vi "Interfaz de caracterizaçao.vi"() -> ()   [LabVIEW 2015]
uses:
  <vilib>/Analysis/baseanly.llb/Mean (DBL).vi
  <instrlib>/Agilent E364X Series/Agilent E364X Series.lvlib
  <instrlib>/Agilent 428X Series/Agilent 428X Series.lvlib
  <vilib>/Analysis/NI_AALBase.lvlib
panel:
  out "Fita2":bool
  out "Fita1":bool
  in  "Passo":dbl=0.01
  out "Fase Med":dbl format="%^.4e"
  in  "Faixa":dbl=2.0
  out "Level":dbl
  out "Config total GA":dbl[](array[numeric])
  out "Final Stop":bool
  in  "error in (no error)":errorcluster
  in  "RLC port":refnum<visa-resource-name>="GPIB0::17::INSTR"
  out "Configuração GA":dbl[](array[numeric])
  out "Otimos":dbl[](array[numeric])
  out "S_ot":dbl
  in  "milliseconds to wait":u32=1000
  out "Returned Data":string
  out "Frec OPT":dbl
  out "H(Oe) OPT":dbl
  out "Bias current OPT":dbl
  out "todo":dbl[](array[numeric])
  out "element":dbl
  out "Iteraciones":i32
  out "Corrente":dbl
  out "RELE 2":bool
  out "Modulo 2":cluster{"X":dbl[], "Y":dbl[]}[](graph) caption="XY Graph"
  out "Fase 2":cluster{"X":dbl[], "Y":dbl[]}[](graph) caption="XY Graph"
  out "Fase":dbl format="%^.4e"
  out "Modulo":dbl format="%^.4e"
  out "Data Status 2":bool=TRUE
  in  "Voltage (V)(1.0V) 2":dbl=1.0 min=0.0 max=20.0 step=0.1 format="%.4f"
  in  "Imp Type (0: CPD)":u32(ring)=15 items=["CPD", "CPQ", "CPG", "CPRP", "CSD", "CSQ", "CSRS", "LPQ", "LPD", "LPG", "LPRP", "LSD", "LSQ", "LSRS", "RX", "ZTD", "ZTR", "GB", "YTD", "YTR"]
  in  "RLC port 2":refnum<visa-resource-name>="GPIB0::17::INSTR"
  in  "error in (no error) 2":errorcluster
  out "RELE":bool
  out "Current Value":dbl
  out "Data Status":bool=TRUE
  in  "Voltage (V)(1.0V)":dbl=1.0 min=0.0 max=20.0 step=0.1 format="%.4f"
  out "Data to MatLab":dbl[](array[numeric])
  out "Data from MatLab":dbl[](array[numeric]) format="%.6g"
  # "Optimization"
  # "Characterization"
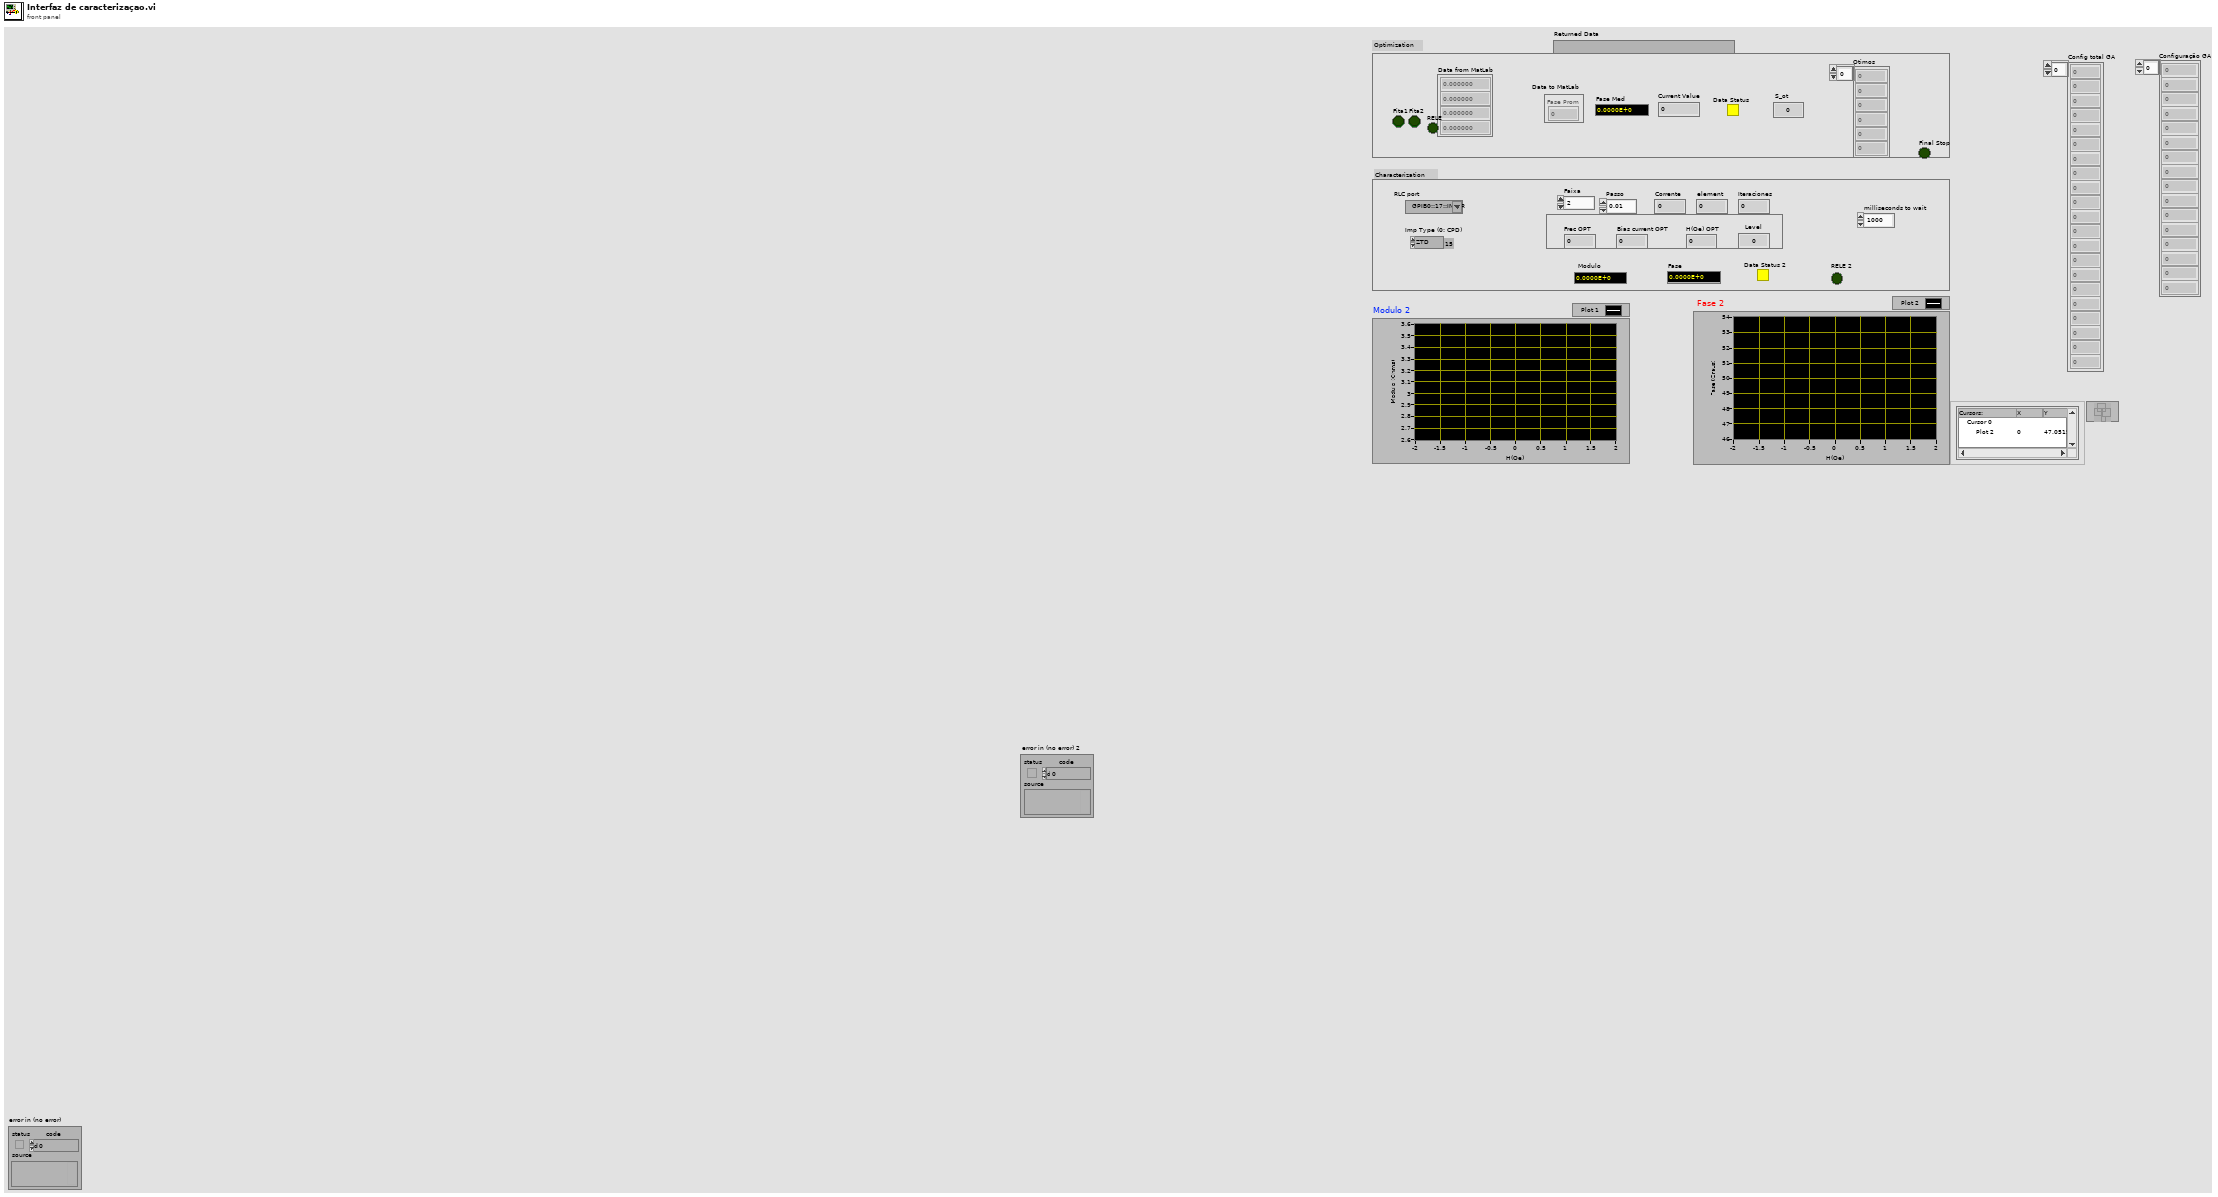
[diagram p1: front panel]
types:
  T1 = enum16{"Standard", "Buffered", "CRLF", "Immediate"}
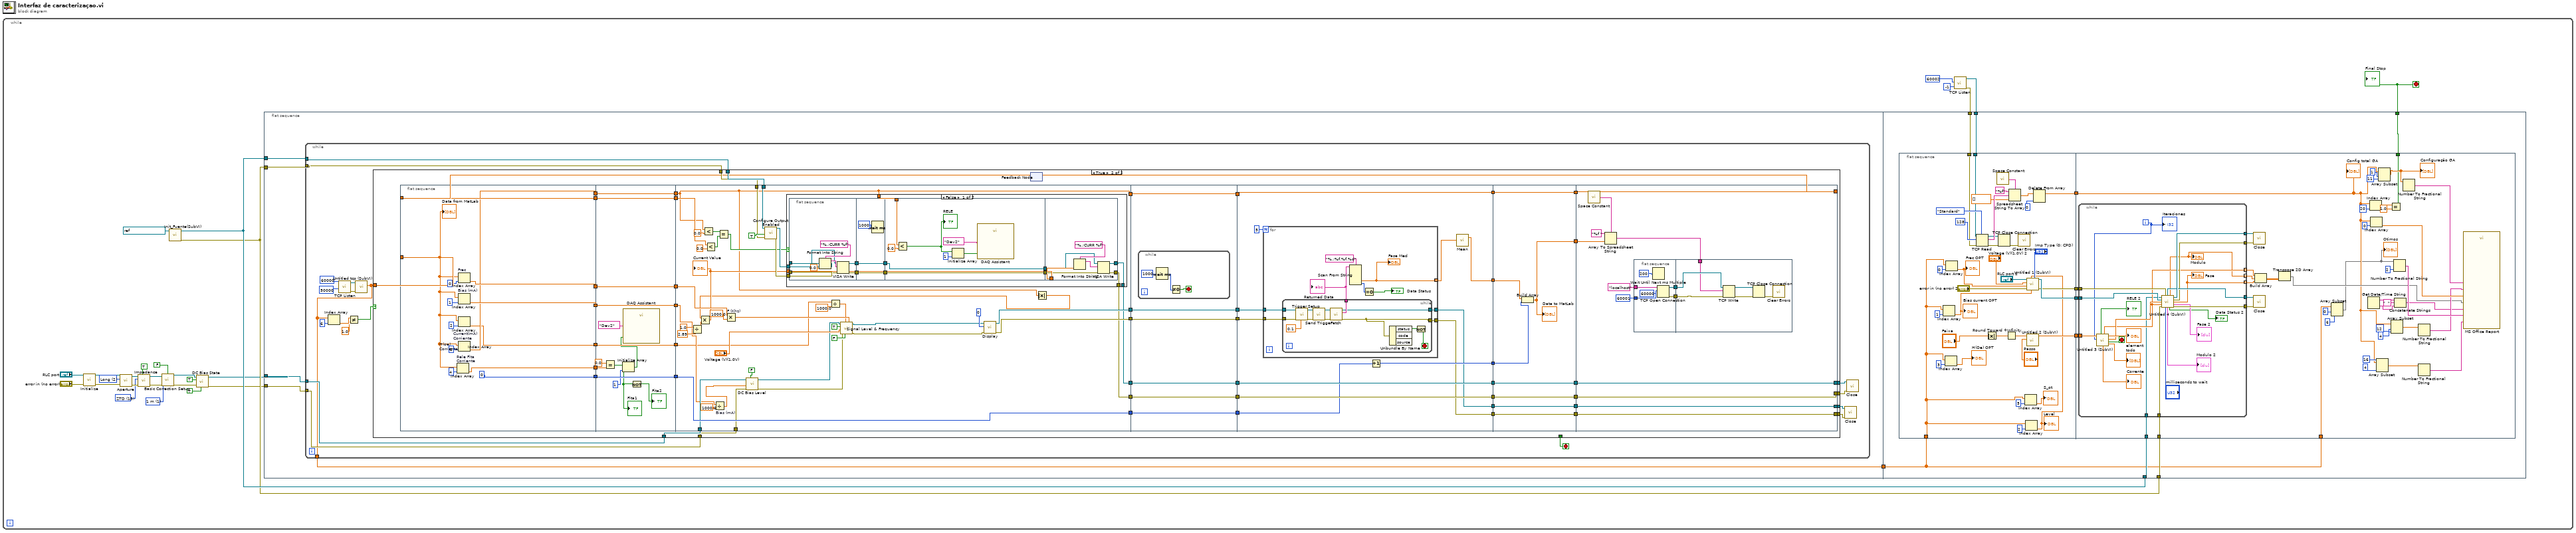
[diagram p0: block diagram]
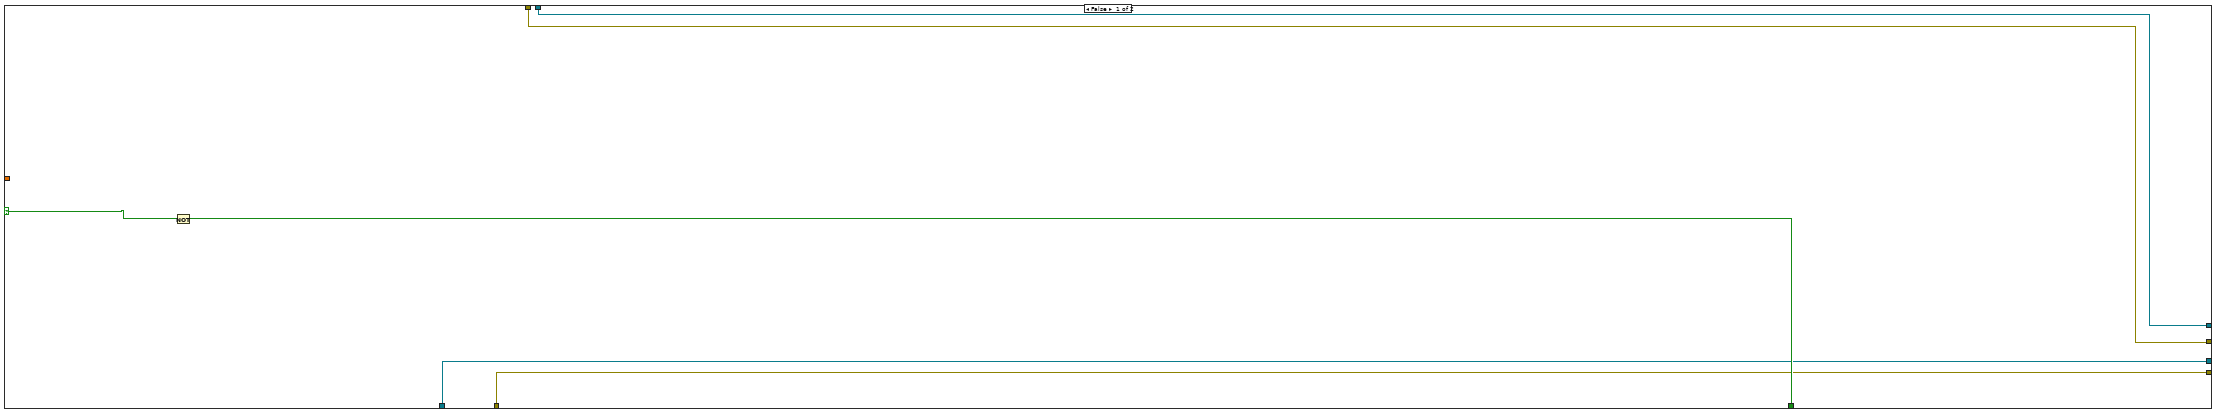
[diagram p2: hidden frame]
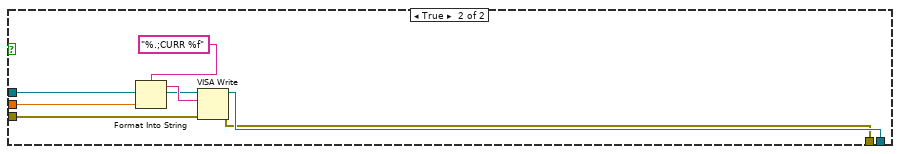
[diagram p3: hidden frame]
diagram:
  n1 = while {
    stop <- w2 stop-if-true
    w13 = u32 1 items=["0 m", "1 m", "2 m", "3 m", "4 m"] ("Cable Length (0: 4 m)")
    w20 = u32 15 items=["CPD", "CPQ", "CPG", "CPRP", "CSD", "CSQ", "CSRS", "LPQ", "LPD", "LPG", "LPRP", "LSD", "LSQ", "LSRS", "RX", "ZTD", "ZTR", "GB", "YTD", "YTR"] ("Imp Type (0: CPD)")
    w24 = u32 2 items=["Short", "Medium", "Long"] ("Integ Time (0: Short)")
    n2 = call <instrlib>:"Initialize.vi"("error in (no error)"="error in (no error)", "VISA resource name"="RLC port") -> ("error out"=w25:errorcluster, "VISA resource name out"=w26:refnum<visa-resource-name>)  [unwired: 8 in]
    n3 = call <instrlib>:"Aperture.vi"("error in (no error)"=w25, "Integ Time (0: Short)"=w24, "VISA resource name"=w26) -> ("error out"=w23:errorcluster, "VISA resource name out"=w22:refnum<visa-resource-name>)  [unwired: 7 in]
    n4 = call <instrlib>:"Impedance.vi"("Auto Range (F: Off)"=TRUE, "error in (no error)"=w23, "Imp Type (0: CPD)"=w20, "VISA resource name"=w22) -> ("error out"=w15:errorcluster, "VISA resource name out"=w17:refnum<visa-resource-name>)  [unwired: 6 in]
    n5 = call <instrlib>:"Basic Correction Setup.vi"("VISA resource name"=w17, "Short Corr (T: On)"=FALSE, "Cable Length (0: 4 m)"=w13, "error in (no error)"=w15) -> ("VISA resource name out"=w16:refnum<visa-resource-name>, "error out"=w14:errorcluster)  [unwired: 9 in, 1 out]
    n6 = call "Init_Fuente(SubVI).vi"("VISA Refnum in"=refnum<visa-resource-name> "GPIB0::5::INSTR") -> ("error out"=w9:errorcluster, "VISA Refnum out"=w10:refnum<visa-resource-name>)  [unwired: 9 in]
    n7 = call <instrlib>:"DC Bias State.vi"("Curr Bias Monitor (F: Off)"=TRUE, "error in (no error)"=w14, "State (F: Off)"=TRUE, "VISA resource name"=w16) -> ("error out"=w7:errorcluster, "VISA resource name out"=w8:refnum<visa-resource-name>)  [unwired: 6 in]
    n8 = flat-sequence {
      tunnel: w10 -> [w33]
      tunnel: w9 -> [w32]
      tunnel: w8 -> [w31]
      tunnel: w7 -> [w30]
      tunnel: [w29] -> w1
      tunnel: w10 -> [w300]
      tunnel: w9 -> [w299]
      tunnel: w4 -> [w297]
      tunnel: w3 -> [w296]
      tunnel: [w295] -> w2
      tunnel: w1 -> [w294]
      frame #0 {
        n9 = while {
          tunnel: w33 -> [w49]
          tunnel: w32 -> [w48]
          tunnel: w31 -> [w51]
          tunnel: w30 -> [w50]
          tunnel: [w38] -> w29
          stop <- w39 stop-if-true
          n10 = call <vilib>:"TCP Listen.vi"("timeout ms (wait forever: -1)"=50000, "port"=u16 60000) -> ("error out"=w44:errorcluster, "connection ID"=w45:refnum<k5>)  [unwired: 5 in, 3 out]
          n11 = call "Untitled tcp (SubVI).vi"("error in (no error)"=w44, "TCP Network Connection in"=w45) -> ("array type (2D Dbl)"=w38:dbl[])  [unwired: 7 in, 2 out]
          n12 = Index Array(array=w38, index=6) -> (element=w42:dbl)
          n13 = Not Equal?(x=w42, y=1.0) -> (x != y?=w40:bool)
          n14 = case shown="True" w40 {
            selector: w40 -> [w57 _]
            tunnel: w51 -> [w55 w81]
            tunnel: w50 -> [w54 w80]
            tunnel: w49 -> [w53 w79]
            tunnel: w48 -> [w52 w78]
            tunnel: w38 -> [_ w76]
            tunnel: [w56 _] -> w39
            tunnel: [w55 w74] -> w37
            tunnel: [w54 w73] -> w36
            tunnel: [w53 w72] -> w35
            tunnel: [w52 w71] -> w34
            frame False {
              n15 = Not(x=w57) -> (.not. x?=w56:bool)
            }
            frame True {
              n16 = flat-sequence {
                tunnel: [w115] -> w70
                tunnel: [w114] -> w68
                tunnel: [0 ("index")] -> w66
                tunnel: [w113] -> w64
                tunnel: [w116] -> w62
                tunnel: w75 -> [w116]
                tunnel: [w110] -> w60
                tunnel: w76 -> [w109]
                tunnel: [w107] -> w58
                tunnel: w70 -> [w132]
                tunnel: [w132] -> w69
                tunnel: w68 -> [w131]
                tunnel: [w131] -> w67
                tunnel: w66 -> [w130]
                tunnel: [w130] -> w65
                tunnel: w64 -> [w129]
                tunnel: [w129] -> w63
                tunnel: w62 -> [w128]
                tunnel: [w128] -> w61
                tunnel: w60 -> [w127]
                tunnel: [w127] -> w59
                tunnel: w58 -> [w126]
                tunnel: w69 -> [w170]
                tunnel: w67 -> [w145]
                tunnel: w65 -> [w162]
                tunnel: [w164] -> w106
                tunnel: [w163] -> w105
                tunnel: [w162] -> w104
                tunnel: [w161] -> w103
                tunnel: [w160] -> w102
                tunnel: w81 -> [w149]
                tunnel: w80 -> [w148]
                tunnel: w79 -> [w157]
                tunnel: w78 -> [w156]
                tunnel: w63 -> [w136]
                tunnel: [w136] -> w101
                tunnel: w61 -> [w137]
                tunnel: w59 -> [w133]
                tunnel: [w224] -> w100
                tunnel: w106 -> [w224]
                tunnel: w105 -> [w223]
                tunnel: [w223] -> w99
                tunnel: w104 -> [w222]
                tunnel: [w222] -> w98
                tunnel: [w221] -> w97
                tunnel: w103 -> [w221]
                tunnel: [w220] -> w96
                tunnel: w102 -> [w220]
                tunnel: w101 -> [w219]
                tunnel: [w219] -> w95
                tunnel: w100 -> [w239]
                tunnel: w99 -> [w228]
                tunnel: w98 -> [w235]
                tunnel: [w233] -> w94
                tunnel: [w229] -> w93
                tunnel: [w238] -> w92
                tunnel: w97 -> [w238]
                tunnel: [w237] -> w91
                tunnel: w96 -> [w237]
                tunnel: [w236] -> w90
                tunnel: [w234] -> w89
                tunnel: w95 -> [w234]
                tunnel: [w230] -> w88
                tunnel: [w268] -> w87
                tunnel: [w266] -> w86
                tunnel: w94 -> [w266]
                tunnel: [w265] -> w85
                tunnel: w93 -> [w265]
                tunnel: [w264] -> w84
                tunnel: w92 -> [w264]
                tunnel: [w263] -> w83
                tunnel: w91 -> [w263]
                tunnel: w90 -> [w262]
                tunnel: [w261] -> w82
                tunnel: w89 -> [w261]
                tunnel: w88 -> [w267]
                tunnel: w87 -> [w274]
                tunnel: [w273] -> w74
                tunnel: w86 -> [w273]
                tunnel: [w272] -> w73
                tunnel: w85 -> [w272]
                tunnel: [w271] -> w72
                tunnel: w84 -> [w271]
                tunnel: [w270] -> w71
                tunnel: w83 -> [w270]
                tunnel: [w269] -> w77
                tunnel: w82 -> [w269]
                frame #0 {
                  n17 = Index Array "Rele Fita\nCorriente"(array=w109, index=4) -> (element=w107:dbl)
                  n18 = Index Array "Frec"(array=w109, index=0) -> (element=w115:dbl)
                  n19 = Index Array "Bias (mA)"(array=w109, index=1) -> (element=w114:dbl)
                  n20 = Index Array "H(oe)\nCorriente"(array=w109, index=3) -> (element=w113:dbl)
                  n21 = Index Array "Current(mA)\nCorriente"(array=w109, index=2) -> (element=w110:dbl)
                  "Data from MatLab" <- w109
                }
                frame #1 {
                  n22 = Equal?(x=0.0, y=w126) -> (x = y?=w121:bool)
                  "Fita1" <- w121
                  n23 = Initialize Array(w121, 1 ("dimension size")) -> (w123:bool[])
                  n24 = call "DAQ Assistant"("data"=w123, "device name"=tag "Dev2") -> ()  [unwired: 16 in, 2 out]
                  n25 = Not(x=w121) -> (.not. x?=→"Fita2":bool)
                }
                frame #2 {
                  n26 = Divide(x=1.0, y=2.89) -> (x/y=w153:dbl)
                  n27 = Less?(x=w136, y=0.0) -> (x < y?=w141:bool)
                  n28 = Less?(x=w137, y=0.0) -> (x < y?=w139:bool)
                  n29 = Divide "Bias (mA)"(x=w145, y=1000.0) -> (x/y=w146:dbl)
                  n30 = Equal?(x=w141, y=w139) -> (x = y?=w138:bool)
                  n31 = Multiply "F (Khz)"(x=w170, y=1000.0) -> (x*y=w169:dbl)
                  n32 = call <instrlib>:"DC Bias Level.vi"("Level Selector (T: Volt)"=FALSE, "error in (no error)"=w148, "Current Level (A) (0.0)"=w146, "VISA resource name"=w149) -> ("error out"=w150:errorcluster, "VISA resource name out"=w151:refnum<visa-resource-name>)  [unwired: 6 in]
                  n33 = call <instrlib>:"Configure Output Enabled.vi"("error in (no error)"=w156, "Output Enabled (F: Off)"=TRUE, "VISA resource name"=w157) -> ("error out"=w172:errorcluster, "VISA resource name out"=w173:refnum<visa-resource-name>)  [unwired: 7 in]
                  n34 = Divide(x=w133, y=1000.0) -> (x/y=w134:dbl)
                  n35 = call <instrlib>:"Signal Level & Frequency.vi"("Frequency Value (Hz) (100KHz)"=w169, "Oscillator Select (T: Voltage)"=FALSE, "Current Level (A) (100uA)"=w134, "error in (no error)"=w150, "Voltage Level (V) (5mV)"="Voltage (V)(1.0V)", "Auto Level Control (F: Off)"=TRUE, "VISA resource name"=w151) -> ("error out"=w158:errorcluster, "VISA resource name out"=w159:refnum<visa-resource-name>)  [unwired: 3 in]
                  n36 = call <instrlib>:"Display.vi"("error in (no error)"=w158, "Display Page (0: Measurement)"=u32 0 ("Display Page (Measurment:0)"), "VISA resource name"=w159) -> ("error out"=w163:errorcluster, "VISA resource name out"=w164:refnum<visa-resource-name>)  [unwired: 7 in]
                  n37 = Absolute Value(x=w136) -> (abs(x)=w143:dbl)
                  n38 = Multiply(x=w143, y=w153) -> (x*y=w152:dbl)
                  "Current Value" <- w152
                  n39 = case shown="False" w138 {
                    tunnel: w173 -> [w186 w216]
                    tunnel: w172 -> [w185 w215]
                    tunnel: [w180 w214] -> w161
                    tunnel: [w181 w213] -> w160
                    tunnel: w152 -> [w182 w212]
                    tunnel: w136 -> [w179 _]
                    frame False {
                      n40 = flat-sequence {
                        tunnel: w186 -> [w188]
                        tunnel: w185 -> [w191]
                        tunnel: [w189] -> w178
                        tunnel: [w187] -> w176
                        tunnel: w178 -> [w196]
                        tunnel: [w196] -> w177
                        tunnel: w176 -> [w195]
                        tunnel: [w195] -> w175
                        tunnel: [w198] -> w184
                        tunnel: w177 -> [w199]
                        tunnel: [w199] -> w183
                        tunnel: w175 -> [w198]
                        tunnel: w179 -> [w197]
                        tunnel: w184 -> [w205]
                        tunnel: w183 -> [w209]
                        tunnel: w182 -> [w208]
                        tunnel: [w207] -> w181
                        tunnel: [w206] -> w180
                        frame #0 {
                          n41 = Format Into String(format string="%.;CURR %f", 0.0 ("input 1")) -> (resulting string=w193:string)  [unwired: 2 in, 1 out]
                          n42 = VISA Write(VISA resource name=w188, write buffer=w193, error in (no error)=w191) -> (VISA resource name out=w187:refnum<visa-resource-name>, error out=w189:errorcluster)  [unwired: 1 out]
                        }
                        frame #1 {
                          n43 = Wait (ms)(milliseconds to wait=u32 1000) -> ()  [unwired: 1 out]
                        }
                        frame #2 {
                          n44 = Less?(x=w197, y=0.0) -> (x < y?=w202:bool)
                          "RELE" <- w202
                          n45 = Initialize Array(w202, 1 ("dimension size")) -> (w200:bool[])
                          n46 = call "DAQ Assistant"("data"=w200, "device name"=tag "Dev2") -> ()  [unwired: 16 in, 2 out]
                        }
                        frame #3 {
                          n47 = Format Into String(format string="%.;CURR %f", w208) -> (resulting string=w211:string)  [unwired: 2 in, 1 out]
                          n48 = VISA Write(VISA resource name=w205, write buffer=w211, error in (no error)=w209) -> (VISA resource name out=w206:refnum<visa-resource-name>, error out=w207:errorcluster)  [unwired: 1 out]
                        }
                      }
                    }
                    frame True {
                      n49 = Format Into String(format string="%.;CURR %f", w212) -> (resulting string=w218:string)  [unwired: 2 in, 1 out]
                      n50 = VISA Write(VISA resource name=w216, write buffer=w218, error in (no error)=w215) -> (VISA resource name out=w214:refnum<visa-resource-name>, error out=w213:errorcluster)  [unwired: 1 out]
                    }
                  }
                }
                frame #3 {
                  n51 = while {
                    stop <- w225 stop-if-true
                    n52 = Wait (ms)(milliseconds to wait=u32 1000) -> (millisecond timer value=w226:u32)
                    n53 = Not Equal To 0?(x=w226) -> (x != 0?=w225:bool)
                  }
                }
                frame #4 {
                  n54 = for {
                    N: 5 -> [_]
                    tunnel: w239 -> [w244]
                    tunnel: [w240] -> w231 mode=indexing
                    tunnel: [w243] -> w233
                    tunnel: [w242] -> w229
                    tunnel: w228 -> [w241]
                    n55 = while {
                      tunnel: [w255] -> w245
                      tunnel: w244 -> [w251]
                      tunnel: [w254] -> w243
                      tunnel: [w253] -> w242
                      tunnel: w241 -> [w252]
                      stop <- w249 stop-if-true
                      n56 = call <instrlib>:"Trigger Setup.vi"("Delay Value (s) (0.0)"=0.1, "error in (no error)"=w252, "VISA resource name"=w251) -> ("error out"=w256:errorcluster, "VISA resource name out"=w257:refnum<visa-resource-name>)  [unwired: 7 in]
                      n57 = call <instrlib>:"Send Trigger.vi"("error in (no error)"=w256, "VISA resource name"=w257) -> ("error out"=w259:errorcluster, "VISA resource name out"=w260:refnum<visa-resource-name>)  [unwired: 8 in]
                      n58 = call <instrlib>:"Fetch.vi"("error in (no error)"=w259, "VISA resource name"=w260) -> ("error out"=w253:errorcluster, "Returned Data"=w255:string, "VISA resource name out"=w254:refnum<visa-resource-name>)  [unwired: 7 in]
                      n59 = Unbundle By Name(w253) -> ("status"=w250:bool)  [unwired: 2 out]
                      n60 = Not(x=w250) -> (.not. x?=w249:bool)
                    }
                    "Returned Data" <- w245
                    n61 = Scan From String(format string="%.;%f,%f,%d", input string=w245) -> (output 2=w240:dbl, output 3=w246:i32)  [unwired: 6 in, 3 out]
                    "Fase Med" <- w240
                    n62 = Equal To 0?(x=w246) -> (x = 0?=→"Data Status":bool)
                  }
                  n63 = Increment(x=w235) -> (x+1=w236:i32)
                  n64 = call-poly <vilib>:"Mean.vi"("X"=w231) -> ("mean"=w230:dbl)  [unwired: 1 out]
                }
                frame #5 {
                  n65 = Build Array(w267, w262) -> (w268:dbl[])
                  "Data to MatLab" <- w268
                }
                frame #6 {
                  n66 = call <vilib>:"Space Constant.vi"() -> ("String"=w280:string)
                  n67 = Array To Spreadsheet String(delimiter (Tab)=w280, array=w274, 3:"%f " ("format string")) -> (spreadsheet string=w275:string)
                  n68 = flat-sequence {
                    tunnel: [w287] -> w278
                    tunnel: [w286] -> w279
                    tunnel: "localhost" ("address") -> [w284]
                    tunnel: u16 60001 ("remote port or service name") -> [w283]
                    tunnel: w279 -> [w289]
                    tunnel: w278 -> [w290]
                    tunnel: w275 -> [w288]
                    frame #0 {
                      n69 = Wait Until Next ms Multiple(millisecond multiple=u32 200) -> ()  [unwired: 1 out]
                      n70 = TCP Open Connection(address=w284, remote port or service name=w283, timeout ms (60000)=60000) -> (connection ID=w287:refnum<k5>, error out=w286:errorcluster)  [unwired: 2 in]
                    }
                    frame #1 {
                      n71 = TCP Write(connection ID=w290, data in=w288, error in (no error)=w289) -> (connection ID out=w292:refnum<k5>, error out=w291:errorcluster)  [unwired: 1 in, 1 out]
                      n72 = TCP Close Connection(connection ID=w292, error in (no error)=w291) -> (error out=w293:errorcluster)  [unwired: 1 in, 1 out]
                      n73 = call <vilib>:"Clear Errors.vi"("error in (no error)"=w293) -> ()  [unwired: 5 in, 2 out]
                    }
                  }
                }
              }
              n74 = feedback #1() -> (w75:dbl)  [unwired: 1 in]
              n75 = feedback-in #1(w77) -> ()
            }
          }
          n76 = call <instrlib>:"Close.vi"("error in (no error)"=w36, "VISA resource name"=w37) -> ()  [unwired: 9 in, 1 out]
          n77 = call <instrlib>:"Close.vi"("error in (no error)"=w34, "VISA resource name"=w35) -> ()  [unwired: 9 in, 1 out]
        }
      }
      frame #1 {
        n78 = flat-sequence {
          tunnel: [w335] -> w303
          tunnel: [w334] -> w302
          tunnel: [w333] -> w301
          tunnel: [w319] -> w298
          tunnel: w297 -> [w318]
          tunnel: w296 -> [w317]
          tunnel: w294 -> [w306]
          tunnel: w303 -> [w378]
          tunnel: w302 -> [w377]
          tunnel: w301 -> [w376]
          tunnel: w300 -> [w371]
          tunnel: w299 -> [w370]
          tunnel: w298 -> [w348]
          tunnel: [w344] -> w295
          tunnel: w294 -> [w341]
          frame #0 {
            n79 = Index Array(array=w306, index=1) -> (element=w310:dbl)
            "Bias current OPT" <- w310
            n80 = Index Array(array=w306, index=3) -> (element=→"H(Oe) OPT":dbl)
            n81 = Index Array(array=w306, index=0) -> (element=w311:dbl)
            "Frec OPT" <- w311
            n82 = TCP Read(connection ID=w318, bytes to read=128, error in (no error)=w317, 7:T1."Standard" ("mode (standard)")) -> (connection ID out=w322:refnum<k5>, data out=w328:string, error out=w323:errorcluster)  [unwired: 1 in]
            n83 = Absolute Value(x="Faixa") -> (abs(x)=w331:dbl)
            n84 = call <vilib>:"Space Constant.vi"() -> ("String"=w320:string)
            n85 = TCP Close Connection(connection ID=w322, error in (no error)=w323) -> (error out=w321:errorcluster)  [unwired: 1 in, 1 out]
            n86 = Round Toward +Infinity(x=w331) -> (ceil(x): smallest int >= x=w332:dbl)
            n87 = Spreadsheet String To Array(delimiter (Tab)=w320, format string="%f", spreadsheet string=w328, array type (2D Dbl)=dbl[] []) -> (array=w329:dbl[])
            n88 = call <vilib>:"Clear Errors.vi"("error in (no error)"=w321) -> ()  [unwired: 5 in, 2 out]
            n89 = Index Array(array=w306, index=5) -> (element=→"S_ot":dbl)
            n90 = Index Array(array=w306, index=2) -> (element=w304:dbl)
            "Level" <- w304
            n91 = call "Untitled 1 (SubVI).vi"("Imp Type (0: CPD)"="Imp Type (0: CPD)", "Bias(mA)"=w310, "Current Level (mA)"=w304, "error in (no error)"="error in (no error) 2", "Frecuency (KHz)"=w311, "Voltage (V)(1.0V)"="Voltage (V)(1.0V) 2", "VISA Refnum in"="RLC port 2") -> ("error out"=w334:errorcluster, "VISA Refnum out"=w335:refnum<visa-resource-name>)  [unwired: 3 in]
            n92 = call "Untitled 2 (SubVI).vi"("Passo"="Passo", "Faixa"=w332) -> ("Array"=w333:dbl[])  [unwired: 9 in]
            n93 = Delete From Array(array=w329, index=0) -> (array with subset deleted=w319:dbl[])  [unwired: 1 in, 1 out]
          }
          frame #1 {
            n94 = while {
              tunnel: [w402] -> w381
              tunnel: [w403] -> w382
              tunnel: [w404] -> w380
              tunnel: [w401] -> w379
              tunnel: w378 -> [w400]
              tunnel: w377 -> [w399]
              tunnel: w376 -> [w398]
              tunnel: [w387] -> w374 mode=indexing
              tunnel: [w386] -> w373 mode=indexing
              tunnel: [w385] -> w372 mode=indexing
              tunnel: w371 -> [w384]
              tunnel: w370 -> [w383]
              i -> [w390]
              stop <- w405 stop-if-true
              n95 = call "Untitled 3 (SubVI).vi"("Numeric 3"=w390, "Array"=w398) -> ("Boolean"=w405:bool, "Numeric"=w388:dbl, "element"=→"element":dbl, "Corrente"=→"Corrente":dbl, "Field"=w387:dbl, "todo"=→"todo":dbl[], "RELE"=→"RELE 2":bool)  [unwired: 3 in]
              n96 = call "Untitled 4 (SubVI).vi"("In source"=w384, "error in RLC"=w399, "RLC in"=w400, "Current"=w388, "Field"=w387, "error in source"=w383, "milliseconds to wait"="milliseconds to wait") -> ("VISA resource name out 2"=w403:refnum<visa-resource-name>, "Modulo 2"=w386:dbl, "VISA Refnum out"=w404:refnum<visa-resource-name>, "error out 3"=w401:errorcluster, "Fase 2"=w385:dbl, "Fase"=→"Fase 2":cluster{"X":dbl[], "Y":dbl[]}[], "Modulo"=→"Modulo 2":cluster{"X":dbl[], "Y":dbl[]}[], "Data Status"=→"Data Status 2":bool, "error out"=w402:errorcluster)
              "Fase" <- w385
              "Modulo" <- w386
              "Iteraciones" <- w390
            }
            n97 = call <instrlib>:"Close.vi"("error in (no error)"=w379, "VISA resource name"=w380) -> ()  [unwired: 9 in, 1 out]
            n98 = call <instrlib>:"Close.vi"("error in (no error)"=w381, "VISA resource name"=w382) -> ()  [unwired: 9 in, 1 out]
            n99 = Build Array(w374, w373, w372) -> (w375:dbl[][])
            n100 = Transpose 2D Array(2D array=w375) -> (transposed array=w353:dbl[][])
            n101 = Array Subset(array=w341, index=0, length=6) -> (w340:dbl[])
            "Otimos" <- w340
            n102 = Get Date/Time String() -> (date string=w369:string, time string=w352:string)  [unwired: 3 in]
            n103 = Index Array(array=w348, index=20) -> (element=w346:dbl)
            n104 = Index Array(array=w348, index=0) -> (element=w357:dbl)
            n105 = Array Subset(array=w348, index=16, length=4) -> (w359:dbl[])
            n106 = Array Subset(array=w348, index=1, length=11) -> (w362:dbl[])
            "Configuração GA" <- w362
            n107 = Equal?(x=w346, y=1.0) -> (x = y?=w344:bool)
            n108 = Array Subset(array=w348, index=12, length=4) -> (w360:dbl[])
            n109 = Number To Fractional String(number=w340, precision (6)=i16 2) -> (F-format string=w356:string[])  [unwired: 2 in]
            n110 = Concatenate Strings(w369, "  " ("string"), w352) -> (w350:string)
            n111 = Number To Fractional String(number=w362) -> (F-format string=w361:string[])  [unwired: 3 in]
            n112 = Number To Fractional String(number=w359) -> (F-format string=w354:string[])  [unwired: 3 in]
            n113 = Number To Fractional String(number=w360) -> (F-format string=w355:string[])  [unwired: 3 in]
            n114 = call "MS Office Report"("Config_GA"=w361, "cross"=w357, "dados"=w353, "Data"=w350, "Lb_Data"=w355, "RLC"=w356, "Ub_Data"=w354) -> ()  [unwired: 19 in, 2 out]
            "Config total GA" <- w348
          }
        }
      }
    }
    n115 = call <vilib>:"TCP Listen.vi"("timeout ms (wait forever: -1)"=-1, "port"=u16 60002) -> ("error out"=w3:errorcluster, "connection ID"=w4:refnum<k5>)  [unwired: 5 in, 3 out]
    "Final Stop" <- w2
  }
